vi "addStatesToQueue.vi"(0 "State(s) in Front (\"\")":string, 5 "State(s) in (\"\")":string, 7 "State(s) at Back (\"\")":string) -> (6 "States Out":string)   [LabVIEW 2019]
panel:
  # "For instructions on how to use the JKI State Machine, examples and video tutorials, visit:\nhttp://jki.net/state-machine/\n\nJKI State Machine™\nhttp://jki.net/state-machine/\nCopyright (C) 2005-2017, JKI <info@jki.net>\nALL RIGHTS RESERVED"
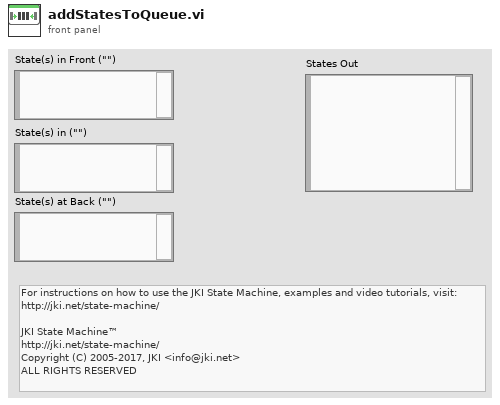
[diagram p1: front panel]
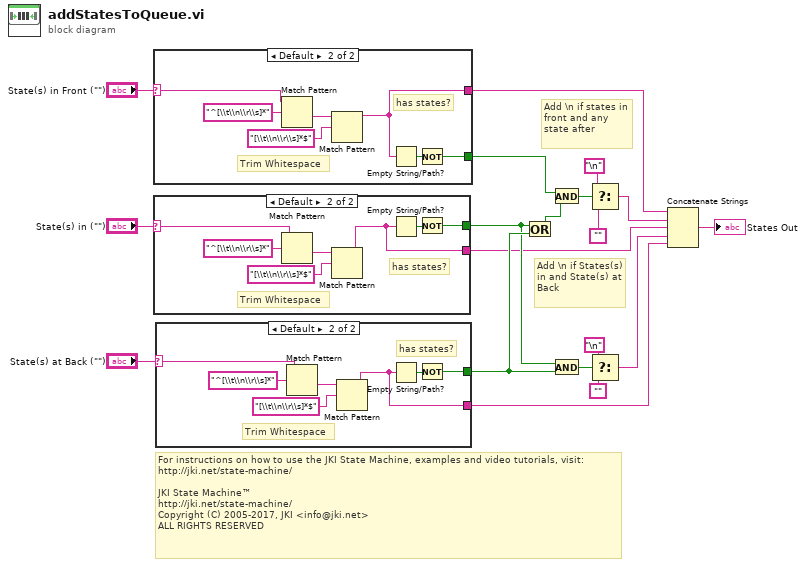
[diagram p0: block diagram]
diagram:
  # "For instructions on how to use the JKI State Machine, examples and video tutorials, visit:\nhttp://jki.net/state-machine/\n\nJKI State Machine™\nhttp://jki.net/state-machine/\nCopyright (C) 2005-2017, JKI <info@jki.net>\nALL RIGHTS RESERVED"
  # "Add \\n if States(s) in and State(s) at Back"
  # "Add \\n if states in front and any state after"
  n1 = case shown="Default" "State(s) in Front (\"\")" {
    selector: "State(s) in Front (\"\")" -> [_ w20]
    tunnel: [_ w25] -> w17
    tunnel: [_ w21] -> w6
    frame "" {
    }
    frame Default {
      # "Trim Whitespace"
      # "has states?"
      n2 = Match Pattern(string=w20, regular expression="^[\\t\\n\\r\\s]*") -> (after substring=w23:string)  [unwired: 1 in, 3 out]
      n3 = Match Pattern(string=w23, regular expression="[\\t\\n\\r\\s]*$") -> (before substring=w21:string)  [unwired: 1 in, 3 out]
      n4 = Empty String/Path?(string/path=w21) -> (empty?=w26:bool)
      n5 = Not(x=w26) -> (.not. x?=w25:bool)
    }
  }
  n6 = case shown="Default" "State(s) in (\"\")" {
    selector: "State(s) in (\"\")" -> [_ w27]
    tunnel: [_ w32] -> w7
    tunnel: [_ w28] -> w5
    frame "" {
    }
    frame Default {
      # "Trim Whitespace"
      # "has states?"
      n7 = Match Pattern(string=w27, regular expression="^[\\t\\n\\r\\s]*") -> (after substring=w30:string)  [unwired: 1 in, 3 out]
      n8 = Match Pattern(string=w30, regular expression="[\\t\\n\\r\\s]*$") -> (before substring=w28:string)  [unwired: 1 in, 3 out]
      n9 = Empty String/Path?(string/path=w28) -> (empty?=w33:bool)
      n10 = Not(x=w33) -> (.not. x?=w32:bool)
    }
  }
  n11 = case shown="Default" "State(s) at Back (\"\")" {
    selector: "State(s) at Back (\"\")" -> [_ w34]
    tunnel: [_ w39] -> w8
    tunnel: [_ w35] -> w4
    frame "" {
    }
    frame Default {
      # "Trim Whitespace"
      # "has states?"
      n12 = Match Pattern(string=w34, regular expression="^[\\t\\n\\r\\s]*") -> (after substring=w37:string)  [unwired: 1 in, 3 out]
      n13 = Match Pattern(string=w37, regular expression="[\\t\\n\\r\\s]*$") -> (before substring=w35:string)  [unwired: 1 in, 3 out]
      n14 = Empty String/Path?(string/path=w35) -> (empty?=w40:bool)
      n15 = Not(x=w40) -> (.not. x?=w39:bool)
    }
  }
  n16 = Or(x=w7, y=w8) -> (x .or. y?=w18:bool)
  n17 = And(x=w17, y=w18) -> (x .and. y?=w16:bool)
  n18 = And(x=w7, y=w8) -> (x .and. y?=w9:bool)
  n19 = Select(t="\n", s=w16, f="") -> (s? t:f=w15:string)
  n20 = Select(t="\n", s=w9, f="") -> (s? t:f=w10:string)
  n21 = Concatenate Strings(w6, w15, w5, w10, w4) -> (→"States Out":string)
